vi "Driver Parse CMD.vi"(8 "Cmd String":string, 11 "Current Driver Index":i32) -> (0 "resulting string":string)   [LabVIEW 2014]
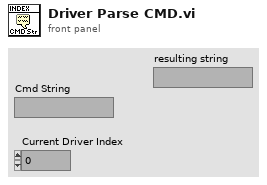
[diagram p1: front panel]
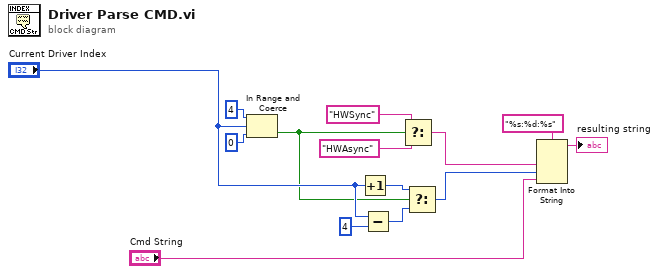
[diagram p0: block diagram]
diagram:
  n1 = In Range and Coerce(upper limit=4, x="Current Driver Index", lower limit=0) -> (In Range?=w8:bool)  [unwired: 1 out]
  n2 = Increment(x="Current Driver Index") -> (x+1=w9:i32)
  n3 = Subtract(x="Current Driver Index", y=4) -> (x-y=w12:i32)
  n4 = Select(t="HWSync" ("format string"), s=w8, f="HWAsync" ("format string")) -> (s? t:f=w7:string)
  n5 = Select(t=w9, s=w8, f=w12) -> (s? t:f=w13:i32)
  n6 = Format Into String(format string="%s:%d:%s", w7, w13, "Cmd String") -> (resulting string=→"resulting string":string)  [unwired: 2 in, 1 out]
